vi "Configure Measurement Characteristics (Transient).vi"(0 "VISA resource name":refnum<visa-resource-name>, 1 "Wideband Frequency Trace Settings":T1={"Frequency Format (1: Hz)"=enum."Hz", "Frequency Reference (0 Hz)"=0.0} {"Frequency Reference (0 Hz)" format="%^#_9g"}, 5 "Phase Unit (0: Deg)":u16(ring) items=["DEG", "GRAD", "RAD"], 7 "Phase X Reference (11.00960 s)":dbl=11.0096 format="%^#_9g", 9 "Enable Wrap Phase (Enable)":bool=TRUE, 11 "error in (no error)":errorcluster, 12 "Narrowband Frequency Trace Settings":T1={"Frequency Format (1: Hz)"=enum."Hz", "Frequency Reference (0 Hz)"=0.0} {"Frequency Reference (0 Hz)" format="%^#_9g"}) -> (4 "VISA resource name out":refnum<visa-resource-name>, 15 "error out":errorcluster)   [LabVIEW 2011, in "Agilent E5052X.lvlib"]
doc: "Configures initial settings for Transient measurement. \n\n<b>Note: </b>\n\nThis VI must be called first before calling \"Configure Measurement(Transient)\" VI."
uses:
  Agilent E5052X.lvlib
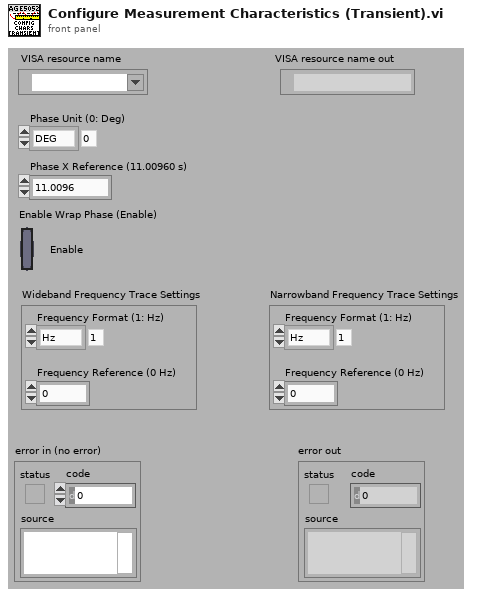
[diagram p1: front panel]
types:
  T1 = cluster{"Frequency Format (1: Hz)":enum16{"DHz", "Hz", "Percent", "ppm"}, "Frequency Reference (0 Hz)":dbl}
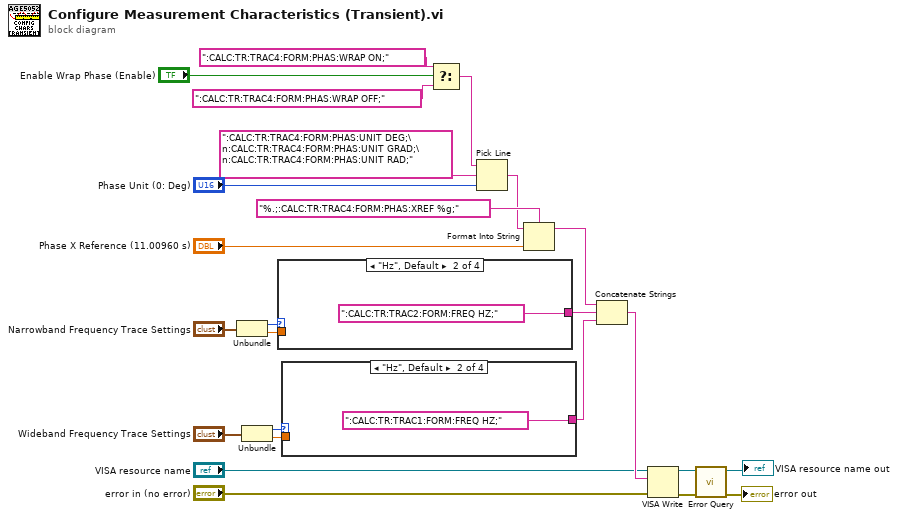
[diagram p0: block diagram]
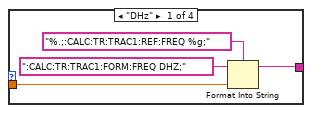
[diagram p2: hidden frame]
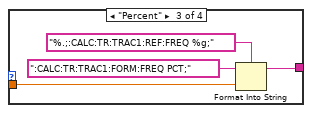
[diagram p3: hidden frame]
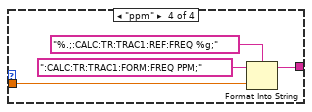
[diagram p4: hidden frame]
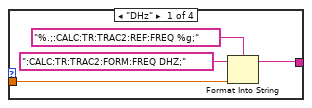
[diagram p5: hidden frame]
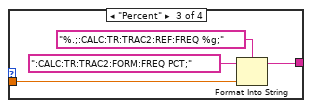
[diagram p6: hidden frame]
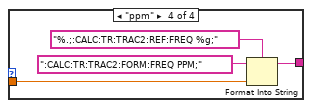
[diagram p7: hidden frame]
diagram:
  n1 = Unbundle("Narrowband Frequency Trace Settings") -> ("Frequency Format (1: Hz)"=w24:enum16{"DHz", "Hz", "Percent", "ppm"}, "Frequency Reference (0 Hz)"=w23:dbl)
  n2 = Unbundle("Wideband Frequency Trace Settings") -> ("Frequency Format (1: Hz)"=w21:enum16{"DHz", "Hz", "Percent", "ppm"}, "Frequency Reference (0 Hz)"=w20:dbl)
  n3 = case shown="\"Hz\", Default" w24 {
    tunnel: w23 -> [w28 _ w31 w35]
    tunnel: [w26 ":CALC:TR:TRAC2:FORM:FREQ HZ;" w32 w36] -> w17
    frame "DHz" {
      n4 = Format Into String(format string="%.;:CALC:TR:TRAC2:REF:FREQ %g;", initial string=":CALC:TR:TRAC2:FORM:FREQ DHZ;", w28) -> (resulting string=w26:string)  [unwired: 1 in, 1 out]
    }
    frame "Hz", Default {
    }
    frame "Percent" {
      n5 = Format Into String(format string="%.;:CALC:TR:TRAC2:REF:FREQ %g;", initial string=":CALC:TR:TRAC2:FORM:FREQ PCT;", w31) -> (resulting string=w32:string)  [unwired: 1 in, 1 out]
    }
    frame "ppm" {
      n6 = Format Into String(format string="%.;:CALC:TR:TRAC2:REF:FREQ %g;", initial string=":CALC:TR:TRAC2:FORM:FREQ PPM;", w35) -> (resulting string=w36:string)  [unwired: 1 in, 1 out]
    }
  }
  n7 = case shown="\"Hz\", Default" w21 {
    tunnel: w20 -> [w41 _ w44 w48]
    tunnel: [w39 ":CALC:TR:TRAC1:FORM:FREQ HZ;" w45 w49] -> w16
    frame "DHz" {
      n8 = Format Into String(format string="%.;:CALC:TR:TRAC1:REF:FREQ %g;", initial string=":CALC:TR:TRAC1:FORM:FREQ DHZ;", w41) -> (resulting string=w39:string)  [unwired: 1 in, 1 out]
    }
    frame "Hz", Default {
    }
    frame "Percent" {
      n9 = Format Into String(format string="%.;:CALC:TR:TRAC1:REF:FREQ %g;", initial string=":CALC:TR:TRAC1:FORM:FREQ PCT;", w44) -> (resulting string=w45:string)  [unwired: 1 in, 1 out]
    }
    frame "ppm" {
      n10 = Format Into String(format string="%.;:CALC:TR:TRAC1:REF:FREQ %g;", initial string=":CALC:TR:TRAC1:FORM:FREQ PPM;", w48) -> (resulting string=w49:string)  [unwired: 1 in, 1 out]
    }
  }
  n11 = Select(t=":CALC:TR:TRAC4:FORM:PHAS:WRAP ON;", s="Enable Wrap Phase (Enable)", f=":CALC:TR:TRAC4:FORM:PHAS:WRAP OFF;") -> (s? t:f=w1:string)
  n12 = Pick Line(string ("")=w1, multi-line string=":CALC:TR:TRAC4:FORM:PHAS:UNIT DEG;\n:CALC:TR:TRAC4:FORM:PHAS:UNIT GRAD;\n:CALC:TR:TRAC4:FORM:PHAS:UNIT RAD;", line index="Phase Unit (0: Deg)") -> (output string=w3:string)
  n13 = Format Into String(format string="%.;:CALC:TR:TRAC4:FORM:PHAS:XREF %g;", initial string=w3, "Phase X Reference (11.00960 s)") -> (resulting string=w2:string)  [unwired: 1 in, 1 out]
  n14 = Concatenate Strings(w2, w17, w16) -> (w11:string)
  n15 = VISA Write(VISA resource name="VISA resource name", write buffer=w11, error in (no error)="error in (no error)") -> (VISA resource name out=w15:refnum<visa-resource-name>, error out=w14:errorcluster)  [unwired: 1 out]
  n16 = call "Error Query.vi"("error in (no error)"=w14, "VISA resource name"=w15) -> ("error out"=→"error out":errorcluster, "VISA resource name out"=→"VISA resource name out":refnum<visa-resource-name>)  [unwired: 6 in, 2 out]
